vi "setDelay.vi"(8 "error in (no error)":errorcluster, 9 "Rate (ps/s)":dbl, 10 "Delay (ps)":dbl, 11 "Instrument.Delay in":refnum<class "Instrument.DelayLine.lvclass">) -> (0 "error out":errorcluster, 3 "Instrument.Delay out":refnum<class "Instrument.DelayLine.lvclass">)   [LabVIEW 2019, in "Instrument.DelayLine.lvclass"]
uses:
  Instrument.DelayLine.lvclass
  Instrument/Instrument.lvclass
  40a8fdee-2d11-416c-bb8b-b04a22bb3818.vi
  Typedefs/setDelay--cluster.ctl
  C:/Users/patrick/Documents/GitHub/Instrument-Framework/lvsrc/Instrument/Instrument.lvclass
  C:/Program Files (x86)/National Instruments/LabVIEW 2019/vi.lib/JKI/JKI SMO/SMO/SMO.lvclass
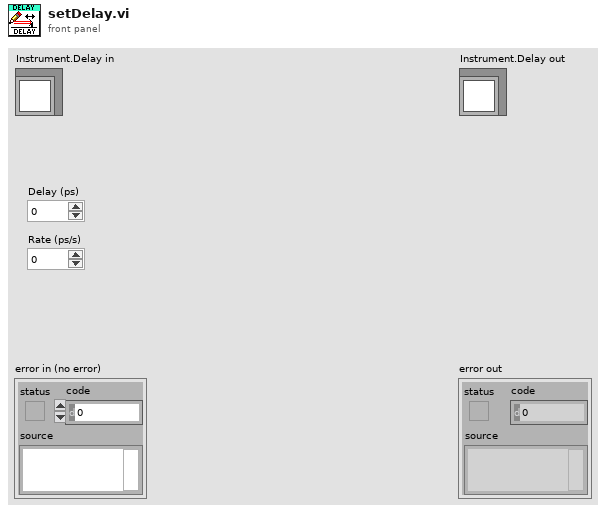
[diagram p1: front panel]
types:
  T1 = typedef "Instrument.DelayLine.lvclass/setDelay--cluster.ctl" = cluster{"Delay":dbl, "Rate":dbl}
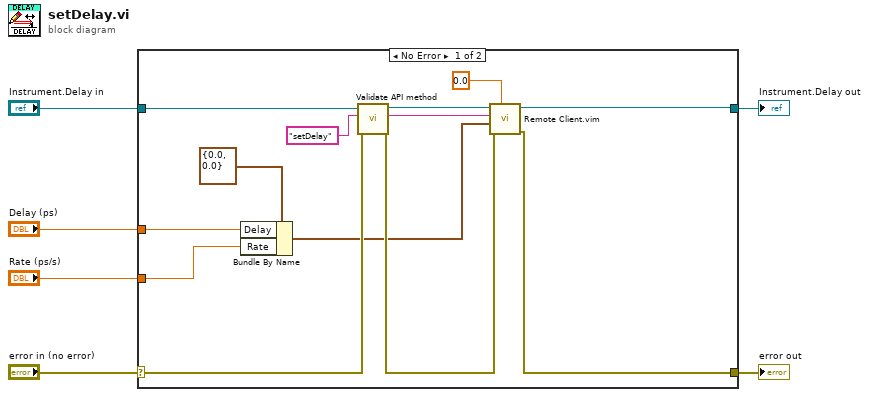
[diagram p0: block diagram]
diagram:
  n1 = case shown="No Error" "error in (no error)" {
    selector: "error in (no error)" -> [w12 w21]
    tunnel: [w13 w21] -> w5
    tunnel: [w14 w20] -> w3
    tunnel: "Instrument.Delay in" -> [w15 w20]
    tunnel: "Delay (ps)" -> [w9 _]
    tunnel: "Rate (ps/s)" -> [w8 _]
    frame No Error {
      n2 = Bundle By Name(cluster=T1 {"Delay"=0.0, "Rate"=0.0} ("setDelay"), "Delay"=w9, "Rate"=w8) -> (w7:T1)
      n3 = call "Validate API method.vi"("error in (no error)"=w12, "command in"="setDelay" ("error message (\"\")"), "Instrument in"=w15) -> ("error out"=w11:errorcluster, "command out"=w17:string, "Instrument out"=w16:refnum<class "Instrument.DelayLine.lvclass">)  [unwired: 6 in]
      n4 = call "Remote Client.vim"("Data Out type"=0.0, "error in (no error)"=w11, "params"=w7, "method"=w17, "Instrument in"=w16) -> ("error out"=w13:errorcluster, "Instrument out"=w14:refnum<class "Instrument.DelayLine.lvclass">)  [unwired: 3 in, 2 out]
    }
    frame Error {
    }
  }
  "error out" <- w5
  "Instrument.Delay out" <- w3
